vi "ref_sys.vi"(3 "error in (no error)":errorcluster, 4 "wr":dbl, 5 "T":dbl) -> (0 "error out":errorcluster, 1 "B":T1, 2 "A":T1)   [LabVIEW 2021]
uses:
  <vilib>/Analysis/Matrix/Datatypes/RealMatrix.ctl
  <vilib>/Analysis/Matrix/Numeric/Multiply/Multiply - RM,R.vi
  <vilib>/Analysis/Matrix/NI_Matrix.lvlib
panel:
  out "aT":dbl
  out "sin(aT)":dbl
  out "cos(aT)":dbl
  out "e^(-aT)":dbl
  out "a":dbl
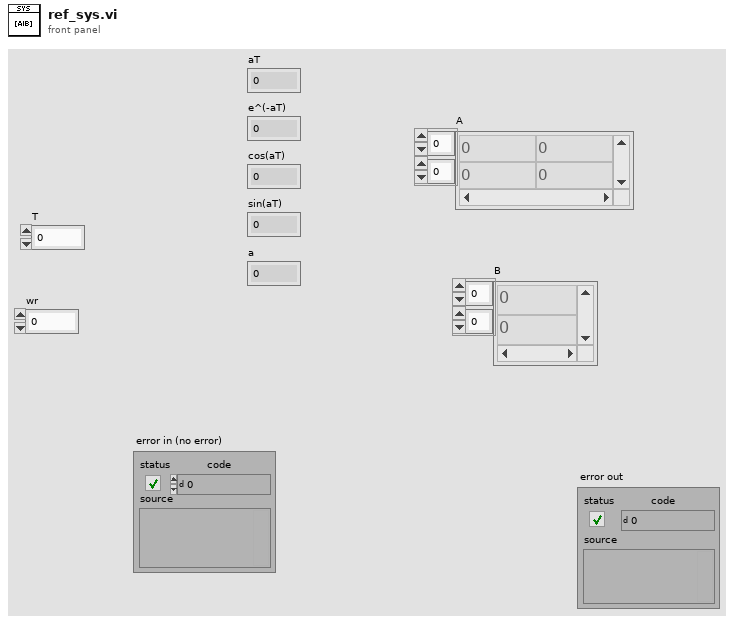
[diagram p1: front panel]
types:
  T1 = typedef "NI_Matrix.lvlib/RealMatrix.ctl" = dbl[][]
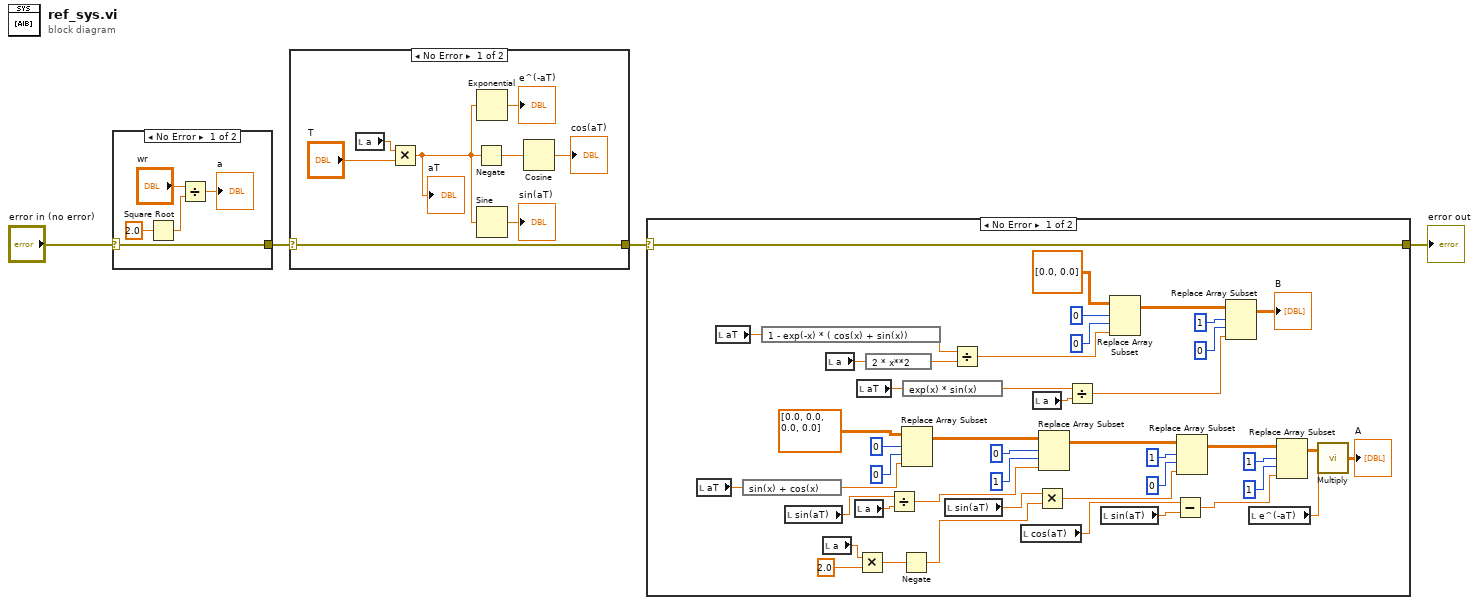
[diagram p0: block diagram]
diagram:
  n1 = case shown="No Error" "error in (no error)" {
    selector: "error in (no error)" -> [w5 w10]
    tunnel: [w5 w10] -> w3
    frame No Error {
      n2 = Square Root(x=2.0) -> (sqrt(x)=w7:dbl)
      n3 = Divide(x="wr", y=w7) -> (x/y=→"a":dbl)
    }
    frame Error {
    }
  }
  n4 = case shown="No Error" w3 {
    selector: w3 -> [w11 w19]
    tunnel: [w11 w19] -> w2
    frame No Error {
      n5 = local read "a"() -> (w16:dbl)
      n6 = Multiply(x=w16, y="T") -> (x*y=w18:dbl)
      "aT" <- w18
      n7 = Negate(x=w18) -> (-x=w17:dbl)
      n8 = Exponential(1:w18) -> (0:→"e^(-aT)":dbl)
      n9 = Sine(x=w18) -> (sin(x)=→"sin(aT)":dbl)
      n10 = Cosine(x=w17) -> (cos(x)=→"cos(aT)":dbl)
    }
    frame Error {
    }
  }
  n11 = case shown="No Error" w2 {
    selector: w2 -> [w59 w66]
    tunnel: [w59 w66] -> w1
    frame No Error {
      n12 = local read "aT"() -> (w24:dbl)
      n13 = local read "aT"() -> (w29:dbl)
      n14 = expression code="sin(x) + cos(x)"(w24) -> (w25:dbl)
      n15 = expression code="1 - exp(-x) * ( cos(x) + sin(x))"(w29) -> (w28:dbl)
      n16 = local read "sin(aT)"() -> (w41:dbl)
      n17 = local read "a"() -> (w35:dbl)
      n18 = local read "a"() -> (w27:dbl)
      n19 = local read "a"() -> (w40:dbl)
      n20 = local read "aT"() -> (w20:dbl)
      n21 = Multiply(x=w35, y=2.0) -> (x*y=w37:dbl)
      n22 = expression code="2 * x**2"(w27) -> (w26:dbl)
      n23 = Divide(x=w41, y=w40) -> (x/y=w42:dbl)
      n24 = Negate(x=w37) -> (-x=w38:dbl)
      n25 = Replace Array Subset(array=dbl[][] [[0.0, 0.0], [0.0, 0.0]], new element=w25, index (row)=0 ("disabled index (row)"), index (col)=0 ("disabled index (col)")) -> (w62:T1)
      n26 = expression code="exp(x) * sin(x)"(w20) -> (w21:dbl)
      n27 = local read "sin(aT)"() -> (w34:dbl)
      n28 = Divide(x=w28, y=w26) -> (x/y=w30:dbl)
      n29 = local read "cos(aT)"() -> (w32:dbl)
      n30 = local read "a"() -> (w22:dbl)
      n31 = Multiply(x=w34, y=w38) -> (x*y=w39:dbl)
      n32 = Replace Array Subset(array=w62, new element=w42, index (row)=0 ("disabled index (row)"), index (col)=1 ("disabled index (col)")) -> (w58:T1)
      n33 = Divide(x=w21, y=w22) -> (x/y=w23:dbl)
      n34 = local read "sin(aT)"() -> (w31:dbl)
      n35 = Replace Array Subset(array=dbl[][] [[0.0], [0.0]], new element=w30, index (row)=0 ("disabled index (row)"), index (col)=0 ("disabled index (col)")) -> (w53:T1)
      n36 = Subtract(x=w32, y=w31) -> (x-y=w33:dbl)
      n37 = Replace Array Subset(array=w58, new element=w39, index (row)=1 ("disabled index (row)"), index (col)=0 ("disabled index (col)")) -> (w55:T1)
      n38 = Replace Array Subset(array=w53, new element=w23, index (row)=1 ("disabled index (row)"), index (col)=0 ("disabled index (col)")) -> (→"B":T1)
      n39 = local read "e^(-aT)"() -> (w43:dbl)
      n40 = Replace Array Subset(array=w55, new element=w33, index (row)=1 ("disabled index (row)"), index (col)=1 ("disabled index (col)")) -> (w45:T1)
      n41 = call-poly <vilib>:"Multiply.vi"("Real Scalar c"=w43, "Real Matrix A"=w45) -> ("A * c"=→"A":T1)
    }
    frame Error {
    }
  }
  "error out" <- w1
